vi "注销设备.vi"(6 "待注销设备MAC":string, 7 "企业数据库":string, 8 "error in (no error)":errorcluster, 11 "数据库引用.i":T1) -> (0 "error out":errorcluster, 3 "数据库引用.o":T1)   [LabVIEW 2013, in "数据库操作.lvclass"]
uses:
  <vilib>/addons/database/Connection.llb/Conn ObjectReference.ctl
  <vilib>/addons/database/Connection.llb/Conn Execute.vi
  <vilib>/addons/database/NI_Database_API.lvlib
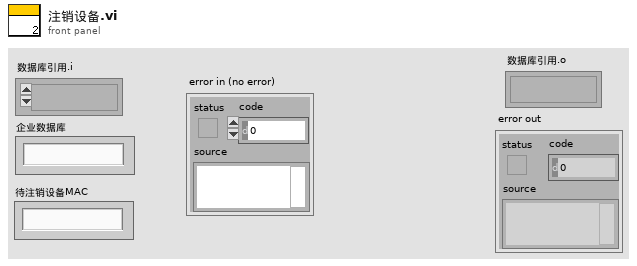
[diagram p1: front panel]
types:
  T1 = typedef "NI_Database_API.lvlib/Conn ObjectReference.ctl" = refnum<k1>
  T2 = enum16{"用户名", "设备MAC", "设备状态", "密码", "职类", "姓名", "电话", "邮箱", "备注", "最后活动"}
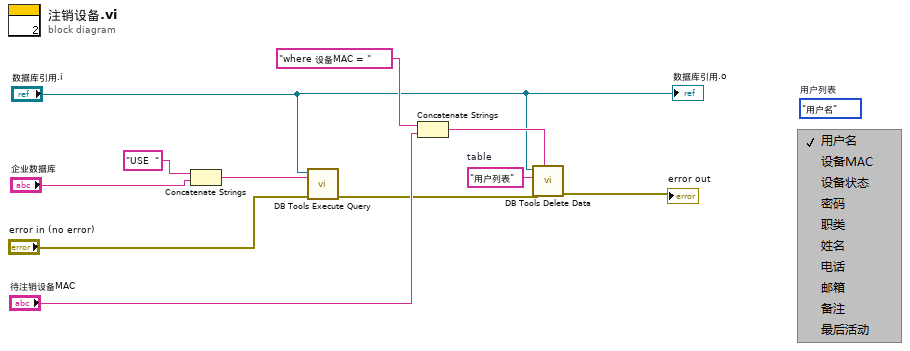
[diagram p0: block diagram]
diagram:
  (unwired) T2."用户名"  # 用户列表
  w7 = "用户列表"  # table
  n1 = Concatenate Strings("USE  " ("字符串"), "企业数据库") -> (w10:string)
  n2 = call-poly <vilib>:"DB Tools Execute Query.vi"("error in (no error)"="error in (no error)", "SQL query"=w10, "connection reference"="数据库引用.i") -> ("error out"=w3:errorcluster)  [unwired: 5 in, 1 out]
  n3 = Concatenate Strings("where 设备MAC = " ("condition"), "待注销设备MAC") -> (w5:string)
  n4 = call <vilib>:"DB Tools Delete Data.vi"("condition"=w5, "error in (no error)"=w3, "table"=w7, "connection reference"="数据库引用.i") -> ("error out"=→"error out":errorcluster)  [unwired: 6 in, 1 out]
  "数据库引用.o" <- "数据库引用.i"
